vi "sequences from string.vi"(8 "error in (no error)":errorcluster, 11 "data to unwrap":string) -> (0 "error out":errorcluster, 3 "sequence definitions":T1[](array[typedef]))   [LabVIEW 2015, in "Simple Sequencer TBM configuration.lvclass"]
uses:
  Simple Sequencer TBM configuration.lvclass
  sequence definition.ctl
  sequencer parent classes/action configuration parent/action configuration.lvclass
  <vilib>/NI/Configuration Framework/serializable configuration/NISE_CEF_serializable configuration.lvclass
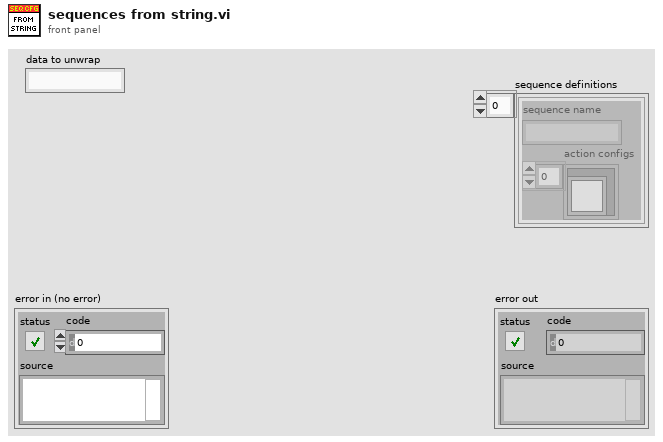
[diagram p1: front panel]
types:
  T1 = typedef "Simple Sequencer TBM configuration.lvclass/sequence definition.ctl" = cluster{"sequence name":string, "action configs":refnum<class "action configuration.lvclass">[]}
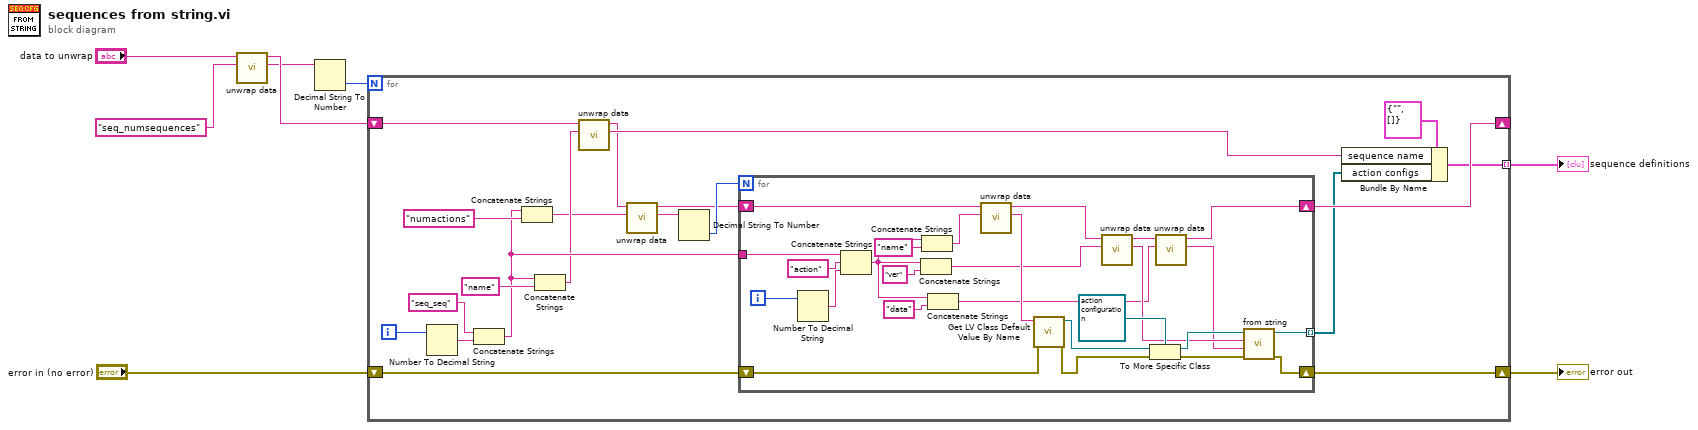
[diagram p0: block diagram]
diagram:
  n1 = call <vilib>:"unwrap data.vi"("identifier"="seq_numsequences", "data to unwrap"="data to unwrap") -> ("unwrapped data"=w2:string, "remaining string"=w4:string)  [unwired: 8 in]
  n2 = Decimal String To Number(string=w2) -> (number=w8:i32)  [unwired: 2 in, 1 out]
  n3 = for {
    N: w8 -> [_]
    shift-right: [w20] -> _
    shift-left: w4 -> [w15]
    shift-right: [w18] -> w5
    shift-left: "error in (no error)" -> [w19]
    tunnel: [w16] -> w6 mode=indexing
    i -> [w27]
    n4 = Number To Decimal String(number=w27) -> (decimal integer string=w28:string)  [unwired: 1 in]
    n5 = Concatenate Strings("seq_seq" ("identifier"), w28) -> (w21:string)
    n6 = Concatenate Strings(w21, "numactions" ("string")) -> (w10:string)
    n7 = Concatenate Strings(w21, "name" ("string")) -> (w14:string)
    n8 = call <vilib>:"unwrap data.vi"("identifier"=w14, "data to unwrap"=w15) -> ("unwrapped data"=w13:string, "remaining string"=w11:string)  [unwired: 8 in]
    n9 = call <vilib>:"unwrap data.vi"("identifier"=w10, "data to unwrap"=w11) -> ("unwrapped data"=w9:string, "remaining string"=w12:string)  [unwired: 8 in]
    n10 = Decimal String To Number(string=w9) -> (number=w22:i32)  [unwired: 2 in, 1 out]
    n11 = for {
      N: w22 -> [_]
      shift-right: [w30] -> w20
      shift-left: w12 -> [w38]
      tunnel: w21 -> [w49]
      shift-right: [w48] -> w18
      shift-left: w19 -> [w44]
      tunnel: [w47] -> w17 mode=indexing
      i -> [w50]
      n12 = Number To Decimal String(number=w50) -> (decimal integer string=w52:string)  [unwired: 1 in]
      n13 = Concatenate Strings(w49, "action" ("string"), w52) -> (w46:string)
      n14 = Concatenate Strings(w46, "ver" ("string")) -> (w34:string)
      n15 = Concatenate Strings(w46, "name" ("string")) -> (w37:string)
      n16 = Concatenate Strings(w46, "data" ("string")) -> (w31:string)
      n17 = call <vilib>:"unwrap data.vi"("identifier"=w37, "data to unwrap"=w38) -> ("unwrapped data"=w36:string, "remaining string"=w35:string)  [unwired: 8 in]
      n18 = call <vilib>:"Get LV Class Default Value By Name.vi"("error in (no error)"=w44, "class name"=w36) -> ("error out"=w43:errorcluster, "object"=w42:refnum<class>)  [unwired: 8 in]
      n19 = call <vilib>:"unwrap data.vi"("identifier"=w34, "data to unwrap"=w35) -> ("unwrapped data"=w33:string, "remaining string"=w32:string)  [unwired: 8 in]
      n20 = To More Specific Class(target class=refnum<class "action configuration.lvclass"> refnum ("shutdown action config"), reference=w42, error in=w43) -> (specific class reference=w39:refnum<class "action configuration.lvclass">, error out=w41:errorcluster)
      n21 = call <vilib>:"unwrap data.vi"("identifier"=w31, "data to unwrap"=w32) -> ("unwrapped data"=w29:string, "remaining string"=w30:string)  [unwired: 8 in]
      n22 = call-dynamic "from string.vi"("error in"=w41, "data"=w29, "version"=w33, "configuration in"=w39) -> ("error out"=w48:errorcluster, "configuration out"=w47:refnum<class "action configuration.lvclass">)  [unwired: 6 in]
    }
    n23 = Bundle By Name(cluster=T1 {"sequence name"="", "action configs"=[]} ("sequence definition"), "sequence name"=w13, "action configs"=w17) -> (w16:T1)
  }
  "sequence definitions" <- w6
  "error out" <- w5
